vi "Init RTTarget.vi"(6 "instVIref":T1, 9 "target structure name":string, 11 "RTTarget in":refnum<class "RTTarget.lvclass">) -> (3 "RTTarget out":refnum<class "RTTarget.lvclass">)   [LabVIEW 2020, in "NI_TargetHelper.lvlib" / "RTTarget.lvclass"]
uses:
  <vilib>/TargetSupport/NI_TargetHelper/RTTarget/RTTarget.lvclass
  <vilib>/TargetSupport/NI_TargetHelper/Instance VIref.ctl
  <vilib>/TargetSupport/NI_TargetHelper/RTTarget/RTTarget.lvclass/RTTarget.ctl
  <vilib>/TargetSupport/NI_TargetHelper/NI_TargetHelper.lvlib
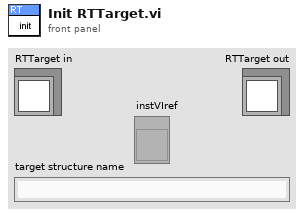
[diagram p1: front panel]
types:
  T1 = typedef "NI_TargetHelper.lvlib/Instance VIref.ctl" = refnum<vi>
  T2 = enum32{"invalid VI type", "Standard VI", "Control VI", "Global VI", "Polymorphic VI", "Configuration VI", "SubSystem", "Facade VI", "Method VI", "Statechart Diagram VI"}
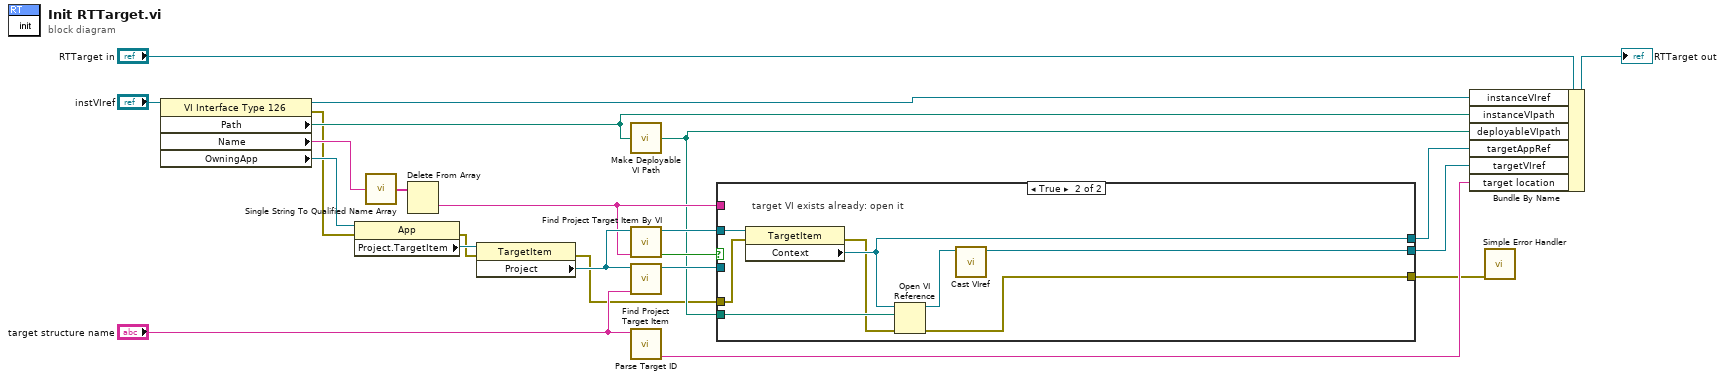
[diagram p0: block diagram]
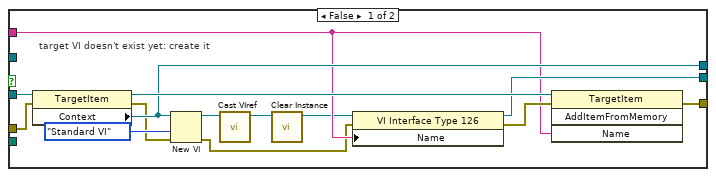
[diagram p2: hidden frame]
diagram:
  n1 = property class="VI Interface Type 126"(reference="instVIref") -> (reference out=w14:T1, error out=w4:errorcluster, "Path"=w12:path, "Name"=w17:string, "OwningApp"=w16:refnum<vi>)  [unwired: 1 in]
  n2 = property class="App"(reference=w16, error in=w4) -> (error out=w3:errorcluster, "Project.TargetItem"=w18:refnum<vi>)  [unwired: 1 out]
  n3 = call <vilib>:"Single String To Qualified Name Array.vi"("Fully Qualified String"=w17) -> ("Fully Qualified Array"=w22:string[])
  n4 = Delete From Array(array=w22) -> (deleted portion=w7:string)  [unwired: 2 in, 1 out]
  n5 = property class="TargetItem"(reference=w18, error in=w3) -> (error out=w2:errorcluster, "Project"=w11:refnum<vi>)  [unwired: 1 out]
  n6 = call <vilib>:"Make Deployable VI Path.vi"("instance path"=w12) -> ("deployable path"=w5:path)
  n7 = call <vilib>:"Find Project Target Item By VI.vi"("vi name"=w7, "project"=w11) -> ("found"=w10:bool, "TargetItem Refnum"=w6:refnum<vi>)  [unwired: 8 in]
  n8 = call <vilib>:"Find Project Target Item.vi"("target structure name"="target structure name", "project"=w11) -> ("TargetItem Refnum"=w15:refnum<vi>)  [unwired: 8 in, 1 out]
  n9 = call <vilib>:"Parse Target ID.vi"("targetID"="target structure name") -> ("target location"=w13:string)  [unwired: 9 in, 1 out]
  n10 = case shown="True" w10 {
    tunnel: w15 -> [w37 _]
    tunnel: w7 -> [w31 _]
    tunnel: [w33 w38] -> w9
    tunnel: [w32 w44] -> w8
    tunnel: w6 -> [_ w45]
    tunnel: w5 -> [_ w43]
    tunnel: w2 -> [w29 w42]
    tunnel: [w24 w40] -> w1
    frame False {
      # "target VI doesn't exist yet: create it"
      n11 = property class="TargetItem"(reference=w37, error in=w29) -> (reference out=w35:refnum<vi>, error out=w28:errorcluster, "Context"=w32:refnum<vi>)
      n12 = New VI(8:w28, 9:T2."Standard VI" ("vi type (standard vi)"), 11:w32) -> (0:w27:errorcluster, 3:w30:refnum<vi>)  [unwired: 4 in]
      n13 = call <vilib>:"Cast VIref.vi"("VI Refnum"=w30) -> ("instVIref"=w26:T1)  [unwired: 10 in]
      n14 = call <vilib>:"Clear Instance.vi"("instVIref"=w26) -> ("instVIref out"=w25:T1)  [unwired: 9 in, 1 out]
      n15 = property class="VI Interface Type 126"(reference=w25, error in=w27, "Name"=w31) -> (reference out=w33:T1, error out=w34:errorcluster)
      n16 = invoke class="TargetItem" method="AddItemFromMemory"(reference=w35, error in=w34, "Name"=w31) -> (error out=w24:errorcluster)  [unwired: 1 in, 3 out]
    }
    frame True {
      # "target VI exists already: open it"
      n17 = property class="TargetItem"(reference=w45, error in=w42) -> (error out=w41:errorcluster, "Context"=w44:refnum<vi>)  [unwired: 1 out]
      n18 = Open VI Reference(application reference (local)=w44, vi path=w43, error in (no error)=w41) -> (vi reference=w39:refnum<vi>, error out=w40:errorcluster)  [unwired: 3 in]
      n19 = call <vilib>:"Cast VIref.vi"("VI Refnum"=w39) -> ("instVIref"=w38:T1)  [unwired: 10 in]
    }
  }
  n20 = Bundle By Name(cluster="RTTarget in", "instanceVIref"=w14, "instanceVIpath"=w12, "deployableVIpath"=w5, "targetAppRef"=w8, "targetVIref"=w9, "target location"=w13) -> (→"RTTarget out":refnum<class "RTTarget.lvclass">)
  n21 = call <vilib>:"Simple Error Handler.vi"("error in (no error)"=w1) -> ()  [unwired: 4 in, 5 out]
